vi "WorkorderHandler_SetActiveOrder.vi"(8 "error in (no error)":errorcluster, 9 "Order":string, 10 "Script":string, 11 "reference":T1) -> (0 "error out":errorcluster, 3 "duplicate reference":T1)   [LabVIEW 2011]
uses:
  DataStructures/WorkorderHandler_ObjectReference.ctl
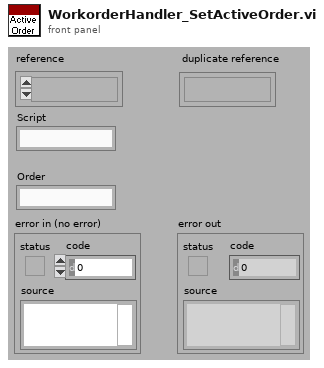
[diagram p1: front panel]
types:
  T1 = typedef "WorkorderHandler_ObjectReference.ctl" = refnum<k1>
  T2 = typedef "WorkorderHandler_ObjectData.ctl" = cluster{"Table":string[][], "Script":string, "Order":string, "No":string, "Time":dbl}
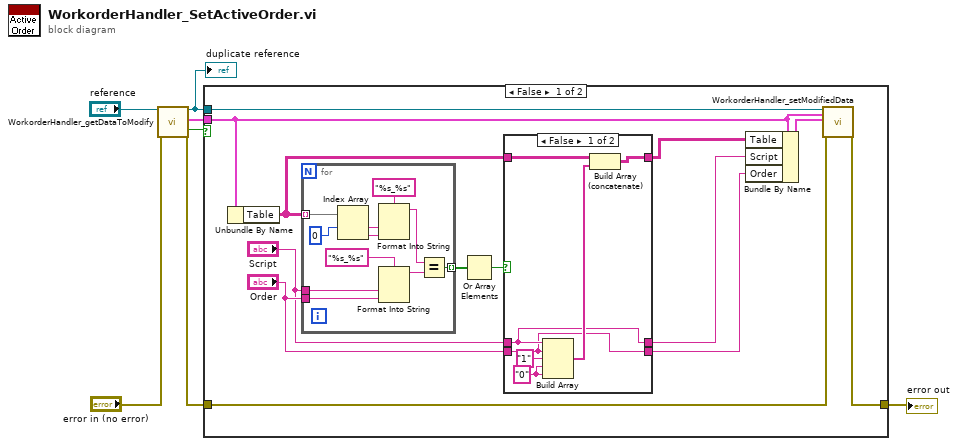
[diagram p0: block diagram]
diagram:
  n1 = call "WorkorderHandler_getDataToModify.vi"("reference"="reference", "error in (no error)"="error in (no error)") -> ("duplicate reference"=w3:T1, "data"=w6:T2, "timed out?"=w1:bool, "error out"=w2:errorcluster)  [unwired: 1 in, 13 out]
  "duplicate reference" <- w3
  n2 = case shown="False" w1 {
    tunnel: [w19 w42] -> w7
    tunnel: w6 -> [w17 _]
    tunnel: w3 -> [w20 _]
    tunnel: w2 -> [w16 w42]
    frame False {
      n3 = Unbundle By Name(w17) -> ("Table"=w12:string[][])
      n4 = for {
        tunnel: w12 -> [w32] mode=indexing
        tunnel: "Script" -> [w36]
        tunnel: "Order" -> [w35]
        tunnel: [w31] -> w15 mode=indexing
        n5 = Index Array(array=w32, index #1=0 ("index")) -> (element #1=w38:string, element #2=w37:string)  [unwired: 1 in]
        n6 = Format Into String(format string="%s_%s", w38, w37) -> (resulting string=w34:string)  [unwired: 2 in, 1 out]
        n7 = Format Into String(format string="%s_%s", w36, w35) -> (resulting string=w33:string)  [unwired: 2 in, 1 out]
        n8 = Equal?(x=w34, y=w33) -> (x = y?=w31:bool)
      }
      n9 = Or Array Elements(Boolean array=w15) -> (logical OR=w14:bool)
      n10 = case shown="False" w14 {
        tunnel: [w25 w30] -> w13
        tunnel: w12 -> [w27 w30]
        tunnel: "Order" -> [w22 w28]
        tunnel: "Script" -> [w23 w29]
        tunnel: [w23 w29] -> w9
        tunnel: [w22 w28] -> w8
        frame False {
          w24 = "0" ("element")
          n11 = Build Array(w23, w22, "1" ("element"), w24, w24) -> (w26:string[])
          n12 = Build Array (concatenate)(w27, w26) -> (w25:string[][])
        }
        frame True {
        }
      }
      n13 = Bundle By Name(cluster=w17, "Table"=w13, "Script"=w9, "Order"=w8) -> (w18:T2)
      n14 = call "WorkorderHandler_setModifiedData.vi"("reference"=w20, "data (unmodified)"=w17, "data"=w18, "error in (no error)"=w16) -> ("error out"=w19:errorcluster)  [unwired: 15 out]
    }
    frame True {
      # "Error or Timed Out"
    }
  }
  "error out" <- w7
